vi "DHE_SetImgState.vi"(2 "DHE_ImgState":T1(ring)) -> ()   [LabVIEW 2016]
uses:
  private/vis/DHE_GBLDriverVariables.vi
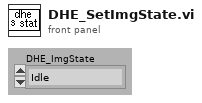
[diagram p1: front panel]
types:
  T1 = enum16{"Idle", "Exposing", "Paused", "AbortExp", "Reading", "AbortRead", "FinishedReading", "Resetting", "Reducing", "Initializing"}
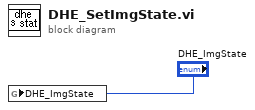
[diagram p0: block diagram]
diagram:
  n1 = global write "DHE_GBLDriverVariables.vi" "DHE_ImgState"("DHE_ImgState") -> ()
